vi "Get Node Reference.vi"(8 "error in (no error)":errorcluster, 10 "name":string, 11 "map reference in":refnum<data-value>) -> (0 "error out":errorcluster, 1 "found?":bool, 2 "node reference":refnum<data-value>, 3 "map reference out":refnum<data-value>)   [LabVIEW 2017, in "NI_Robotics_DirectedGraphWorldMap.lvclass"]
doc: "Returns a reference to the map node you specify."
uses:
  <vilib>/robotics/Navigation/shared/WorldMap/DirectedGraphWorldMap/NI_Robotics_DirectedGraphWorldMap.lvclass
  <vilib>/robotics/Navigation/shared/MapNode/DirectedGraphMapNode/NI_Robotics_DirectedGraphMapNode.lvclass
  <vilib>/robotics/Navigation/shared/WorldMap/DirectedGraphWorldMap/NI_Robotics_DirectedGraphWorldMap.lvclass/NI_Robotics_DirectedGraphWorldMap.ctl
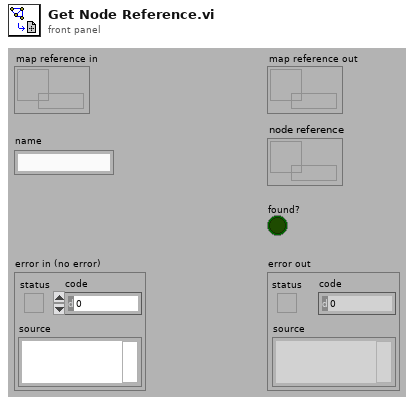
[diagram p1: front panel]
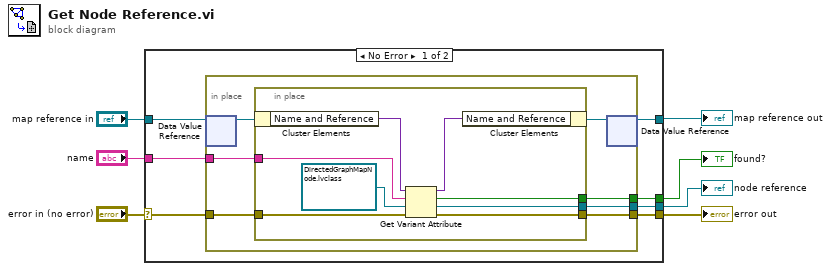
[diagram p0: block diagram]
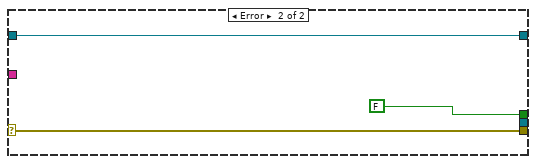
[diagram p2: hidden frame]
diagram:
  n1 = case shown="No Error" "error in (no error)" {
    selector: "error in (no error)" -> [w11 w32]
    tunnel: [w10 w32] -> w6
    tunnel: "name" -> [w14 _]
    tunnel: [w13 FALSE] -> w4
    tunnel: [w12 _] -> w3
    tunnel: "map reference in" -> [w9 w30]
    tunnel: [w8 w30] -> w1
    frame No Error {
      n2 = in-place {
        in-place-border: w14 -> [w21]
        in-place-border: [w20] -> w13
        in-place-border: [w19] -> w12
        in-place-border: w11 -> [w18]
        in-place-border: [w17] -> w10
        n3 = in-place-dvr #1(w9) -> (w16:refnum<class "NI_Robotics_DirectedGraphWorldMap.lvclass">)  [unwired: 1 out]
        n4 = in-place {
          in-place-border: w21 -> [w27]
          in-place-border: [w26] -> w20
          in-place-border: [w24] -> w19
          in-place-border: w18 -> [w23]
          in-place-border: [w22] -> w17
          n5 = in-place-cluster #2(w16) -> ("Name and Reference"=w29:variant)
          n6 = Get Variant Attribute(Variant=w29, name=w27, default value (empty Variant)=refnum<data-value> refnum ("Node ref"), error in=w23) -> (duplicate Variant=w28:variant, found=w26:bool, value=w24:refnum<data-value>, error out=w22:errorcluster)
          n7 = in-place-cluster #2("Name and Reference"=w28) -> (w15:refnum<class "NI_Robotics_DirectedGraphWorldMap.lvclass">)
        }
        n8 = in-place-dvr #1(w15) -> (w8:refnum<data-value>)  [unwired: 1 out]
      }
    }
    frame Error {
    }
  }
  "error out" <- w6
  "node reference" <- w3
  "found?" <- w4
  "map reference out" <- w1
